vi "Save Config File.vi"(10 "base path":path) -> (1 "Cancel":bool, 2 "new file name":string)   [LabVIEW 2018]
panel:
  out "布尔":bool
  in  "退出":bool
  in  "Bar":bool
  in  "H/W Config File List":i32(listbox)
  in  "Boolean":bool
  in  "Cancel":bool
  in  "OK":bool
  in  "H/W Config File Name(*.hwc)":string
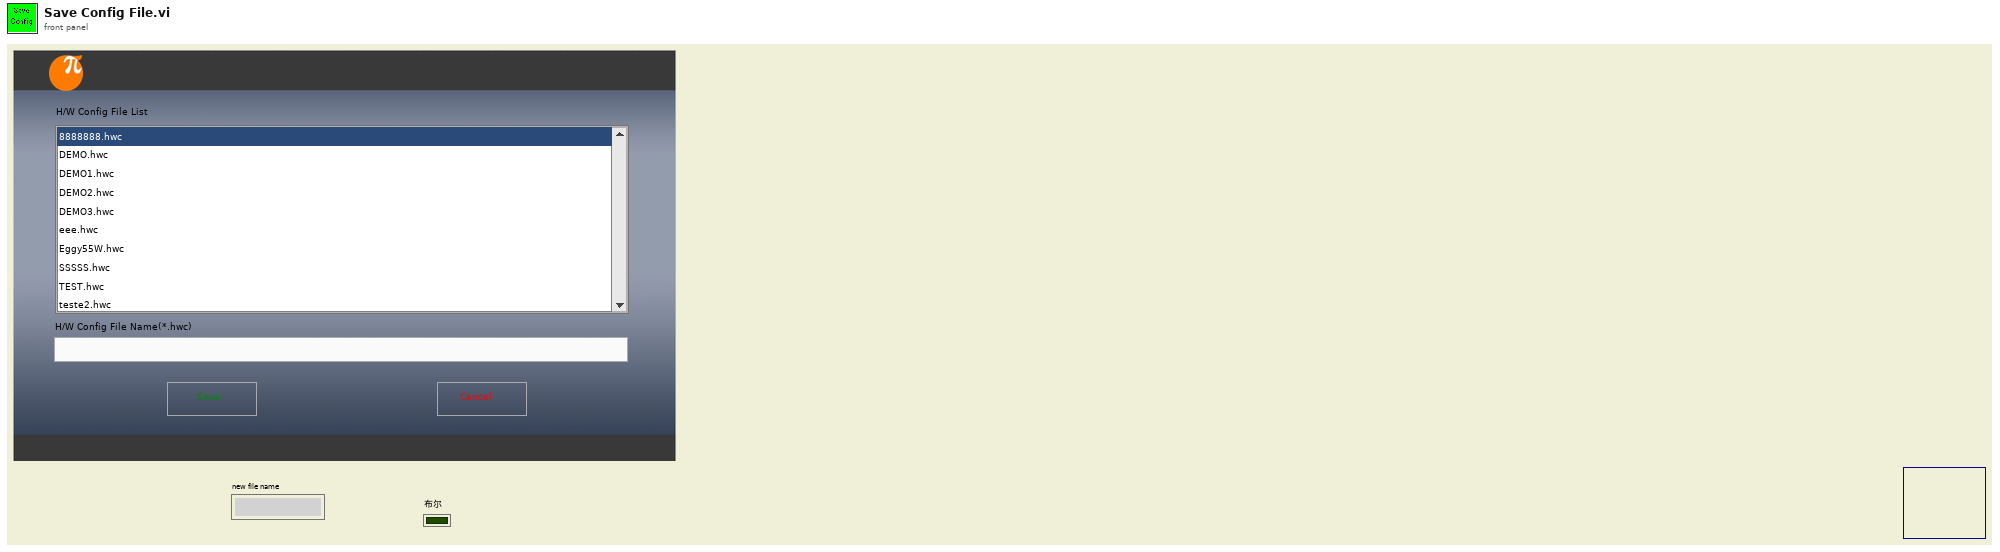
[diagram p1: front panel]
types:
  T1 = typedef "Window Refnum.ctl" = refnum<k1>
  T2 = typedef "Window Rectangle.ctl" = cluster{"left":i16, "top":i16, "right":i16, "bottom":i16}
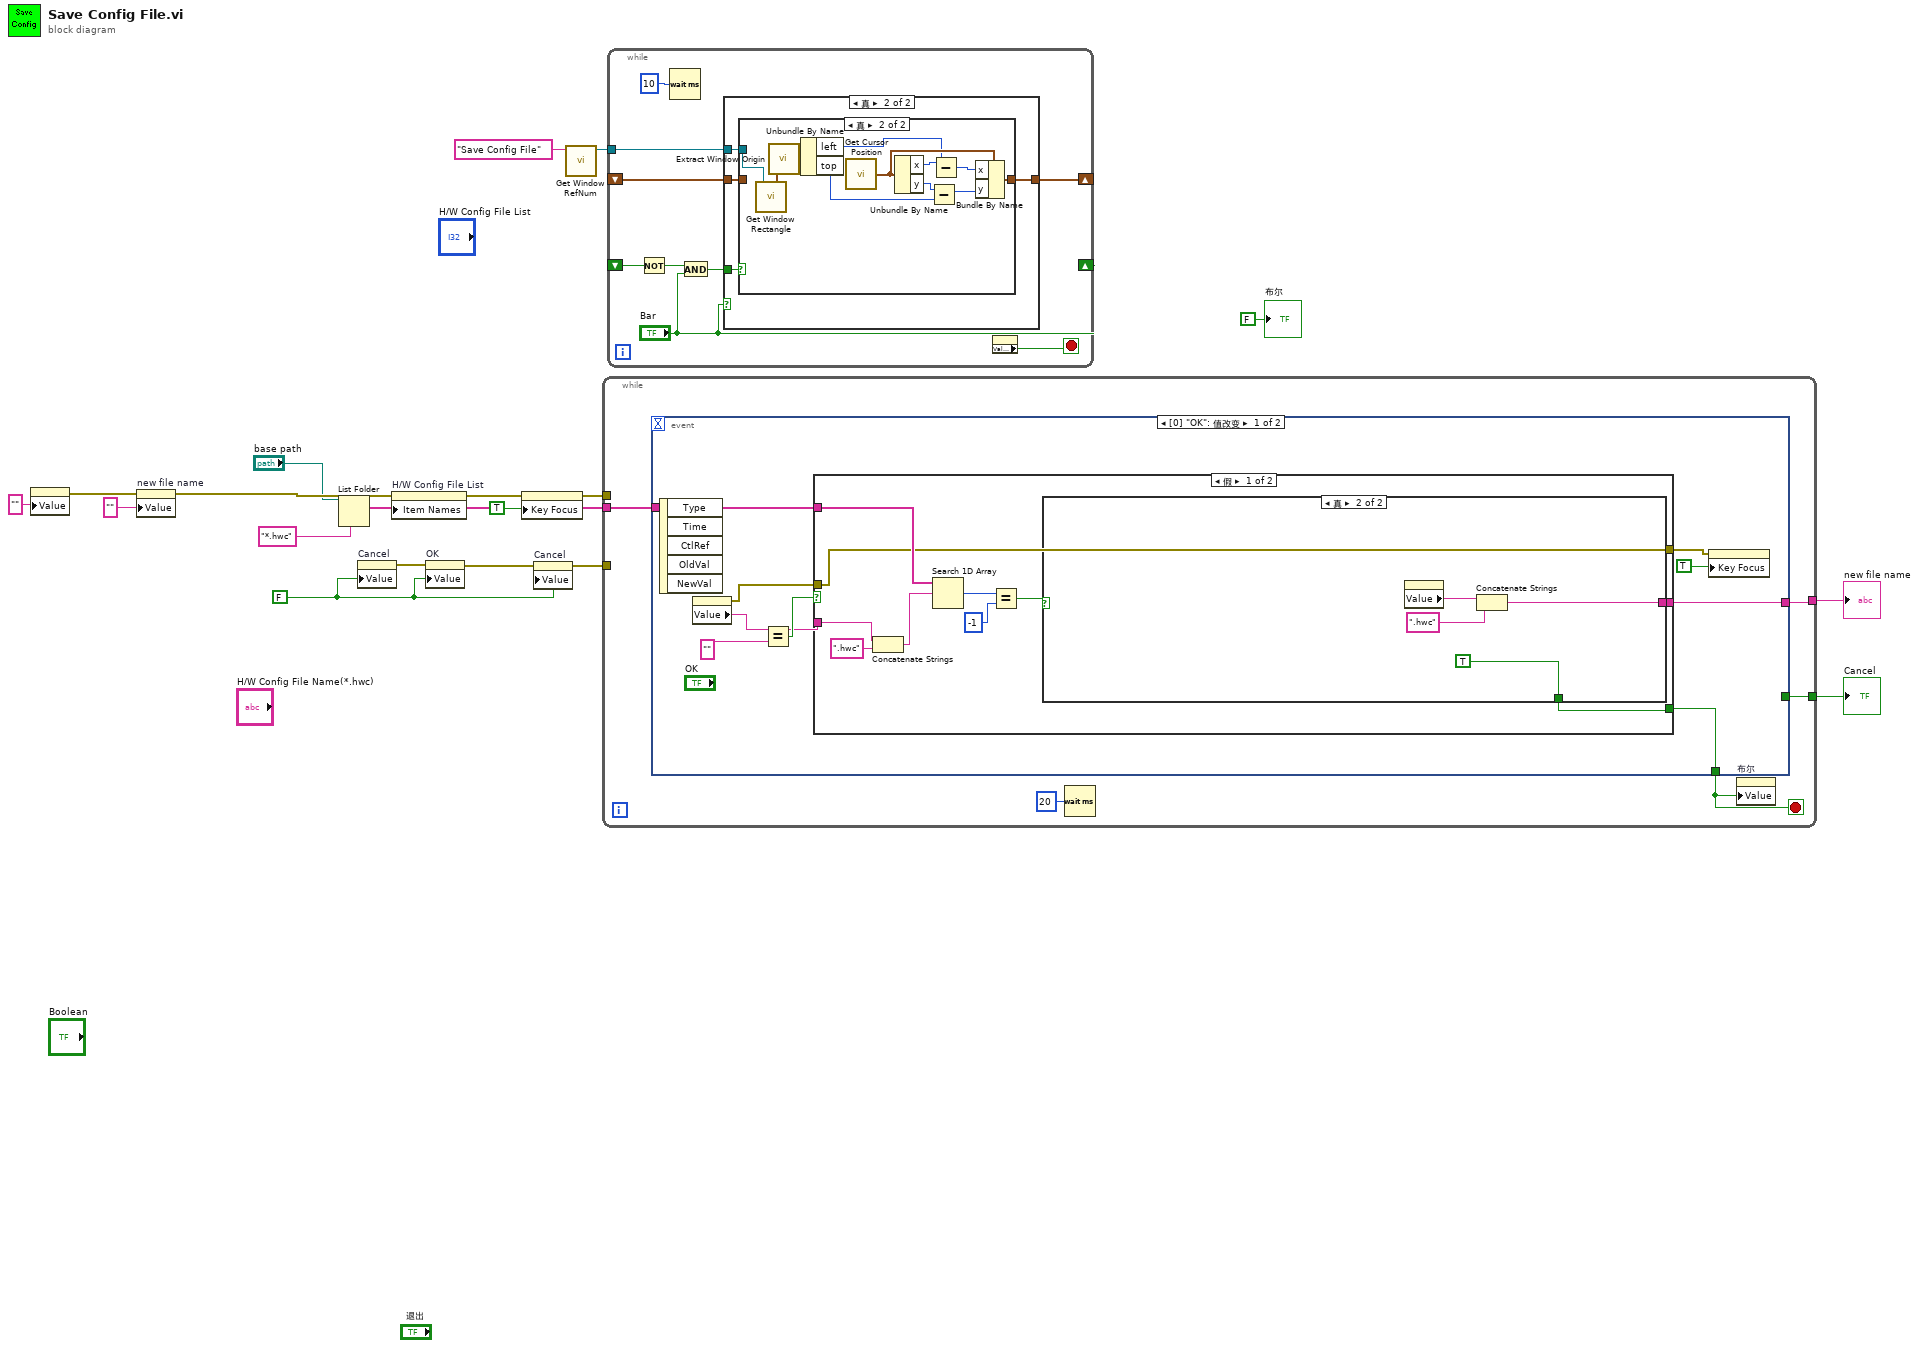
[diagram p0: block diagram]
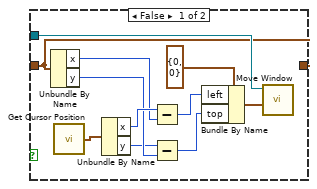
[diagram p3: hidden frame]
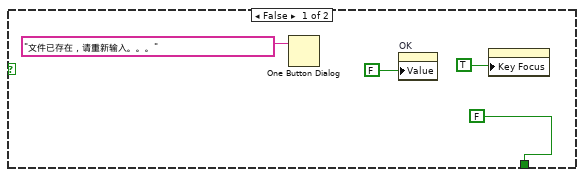
[diagram p4: hidden frame]
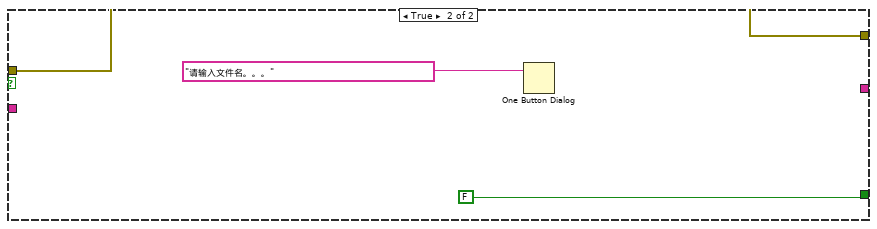
[diagram p5: hidden frame]
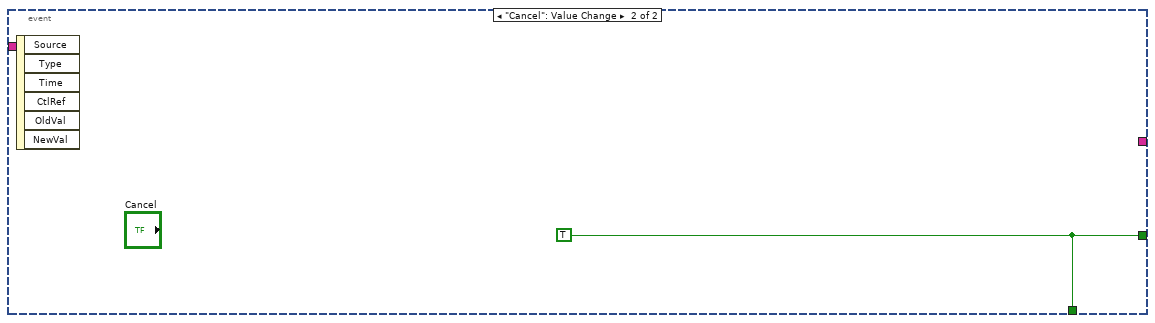
[diagram p6: hidden frame]
diagram:
  w11 = FALSE
  n1 = property on="H/W Config File Name(*.hwc)" class="Str"("Value"="" ("H/W Config File Name(*.hwc)")) -> (error out=w5:errorcluster)  [unwired: 2 in, 1 out]
  n2 = property on="new file name" class="Str"(error in=w5, "Value"="") -> (error out=w8:errorcluster)  [unwired: 1 in, 1 out]
  n3 = List Folder(path="base path", pattern="*.hwc") -> (filenames=w10:string[])  [unwired: 1 in, 4 out]
  n4 = property on="Cancel" class="Bool (严格)"("Value"=w11) -> (error out=w13:errorcluster)  [unwired: 2 in, 1 out]
  n5 = property on="H/W Config File List" class="LstBox (严格)"(error in=w8, "Item Names"=w10) -> (error out=w16:errorcluster)  [unwired: 1 in, 1 out]
  n6 = property on="OK" class="Bool (严格)"(error in=w13, "Value"=w11) -> (error out=w12:errorcluster)  [unwired: 1 in, 1 out]
  n7 = property on="H/W Config File Name(*.hwc)" class="Str"(error in=w16, "Key Focus"=TRUE) -> (error out=w18:errorcluster)  [unwired: 1 in, 1 out]
  n8 = property on="Cancel" class="Bool (严格)"(error in=w12, "Value"=w11) -> (error out=w14:errorcluster)  [unwired: 1 in, 1 out]
  n9 = call "Get Window RefNum.vi"("window name (\"\")"="Save Config File" ("window name (\"\")")) -> ("window refnum (NaWR)"=w2:T1)  [unwired: 1 in, 7 out]
  n10 = while {
    tunnel: w18 -> [_]
    tunnel: [w23] -> w15
    tunnel: w14 -> [_]
    tunnel: w10 -> [w22]
    tunnel: [w21] -> w9
    stop <- w20 stop-if-true
    n11 = event shown="[0] \"OK\": 值改变" {
      selector: _ -> [_ _]
      dyn-events: _ -> [_ _]
      timeout: _ -> [_ _]
      tunnel: [w33 w55] -> w20
      tunnel: [_ w55] -> w23
      tunnel: w22 -> [w32 _]
      tunnel: [w31 _] -> w21
      event "OK": Value Change {
        n12 = event-data() -> ()  [unwired: 6 out]
        n13 = property on="H/W Config File Name(*.hwc)" class="Str"() -> (error out=w26:errorcluster, "Value"=w28:string)  [unwired: 2 in, 1 out]
        n14 = Equal?(x=w28, y="") -> (x = y?=w29:bool)
        n15 = case shown="假" w29 {
          tunnel: [w36 FALSE] -> w33
          tunnel: w28 -> [w43 _]
          tunnel: w32 -> [w40 _]
          tunnel: [w35 _] -> w31
          tunnel: w26 -> [w34 w53]
          tunnel: [w34 w53] -> w25
          frame False {
            n16 = Concatenate Strings(w43, ".hwc" ("string")) -> (w41:string)
            n17 = Search 1D Array(1D array=w40, element=w41) -> (index of element=w39:i32)  [unwired: 1 out]
            n18 = Equal?(x=w39, y=-1) -> (x = y?=w37:bool)
            n19 = case shown="真" w37 {
              tunnel: [FALSE TRUE] -> w36
              tunnel: [_ w49] -> w35
              frame False {
                n20 = One Button Dialog(message="文件已存在，请重新输入。。。" ("IP Text")) -> ()  [unwired: 1 in, 1 out]
                n21 = property on="OK" class="Bool (严格)"("Value"=FALSE) -> ()  [unwired: 2 in, 2 out]
                n22 = property on="H/W Config File Name(*.hwc)" class="Str"("Key Focus"=TRUE) -> ()  [unwired: 2 in, 2 out]
              }
              frame True {
                n23 = property on="H/W Config File Name(*.hwc)" class="Str"() -> ("Value"=w50:string)  [unwired: 2 in, 2 out]
                n24 = Concatenate Strings(w50, ".hwc") -> (w49:string)
              }
            }
          }
          frame True {
            n25 = One Button Dialog(message="请输入文件名。。。" ("IP Text")) -> ()  [unwired: 1 in, 1 out]
          }
        }
        n26 = property on="H/W Config File Name(*.hwc)" class="Str"(error in=w25, "Key Focus"=TRUE) -> ()  [unwired: 1 in, 2 out]
      }
      event "Cancel": Value Change {
        w55 = TRUE
        n27 = event-data() -> ()  [unwired: 7 out]
      }
    }
    n28 = Wait (ms)(milliseconds to wait=u32 20) -> ()  [unwired: 1 out]
    n29 = property on="布尔" class="Bool (严格)"("Value"=w20) -> ()  [unwired: 2 in, 2 out]
  }
  "Cancel" <- w15
  "new file name" <- w9
  n30 = while {
    shift-left: _ -> [w58]
    shift-right: [w59] -> _
    shift-left: _ -> [w62]
    shift-right: ["Bar"] -> _
    tunnel: w2 -> [w63]
    stop <- w56 stop-if-true
    n31 = Not(x=w62) -> (.not. x?=w61:bool)
    n32 = Wait (ms)(milliseconds to wait=u32 10) -> ()  [unwired: 1 out]
    n33 = And(x=w61, y="Bar") -> (x .and. y?=w57:bool)
    n34 = case shown="真" "Bar" {
      tunnel: w63 -> [_ w69]
      tunnel: [w65 w68] -> w59
      tunnel: w58 -> [w65 w66]
      tunnel: w57 -> [_ w67]
      frame False {
      }
      frame True {
        n35 = case shown="真" w67 {
          tunnel: w69 -> [w75 w91]
          tunnel: [w70 w81] -> w68
          tunnel: w66 -> [w70 _]
          frame False {
            n36 = Unbundle By Name(w70) -> ("x"=w78:i16, "y"=w77:i16)
            n37 = call "Get Cursor Position.vi"() -> ("cursor position"=w80:cluster{"x":i16, "y":i16})
            n38 = Unbundle By Name(w80) -> ("x"=w79:i16, "y"=w76:i16)
            n39 = Subtract(x=w79, y=w78) -> (x-y=w72:i16)
            n40 = Subtract(x=w76, y=w77) -> (x-y=w73:i16)
            n41 = Bundle By Name(cluster=cluster{"left":i16, "top":i16} {"left"=0, "top"=0} ("new position (0,0)"), "left"=w72, "top"=w73) -> (w71:cluster{"left":i16, "top":i16})
            n42 = call "Move Window.vi"("new position (0,0)"=w71, "window refnum (NaWR)"=w75) -> ()  [unwired: 2 in, 4 out]
          }
          frame True {
            n43 = call "Get Window Rectangle.vi"("window refnum (NaWR)"=w91) -> ("window rect"=w90:T2)  [unwired: 1 in, 5 out]
            n44 = call "Extract Window Origin.vi"("window rect"=w90) -> ("window origin"=w89:cluster{"left":i16, "top":i16})  [unwired: 1 out]
            n45 = Unbundle By Name(w89) -> ("left"=w86:i16, "top"=w85:i16)
            n46 = call "Get Cursor Position.vi"() -> ("cursor position"=w88:cluster{"x":i16, "y":i16})
            n47 = Unbundle By Name(w88) -> ("x"=w87:i16, "y"=w84:i16)
            n48 = Subtract(x=w84, y=w85) -> (x-y=w83:i16)
            n49 = Subtract(x=w87, y=w86) -> (x-y=w82:i16)
            n50 = Bundle By Name(cluster=w88, "x"=w82, "y"=w83) -> (w81:cluster{"x":i16, "y":i16})
          }
        }
      }
    }
    n51 = property on="布尔" class="Bool (严格)"() -> ("Value"=w56:bool)  [unwired: 2 in, 2 out]
  }
  "布尔" <- FALSE ("布尔")
